vi "Get Physical DMA Address.vi"(8 "error in (no error)":errorcluster, 10 "Address2":u32, 11 "Address1":u32) -> (0 "error out":errorcluster, 1 "function return":u32, 2 "Address2 out":u32, 3 "Address1 out":u32)   [LabVIEW 2014, in "atmcd32d.lvlib"]
doc: "unsigned int WINAPI GetPhysicalDMAAddress(unsigned long * Address1, unsigned long * Address2);"
uses:
  atmcd32d.lvlib
  atmcd32d.dll
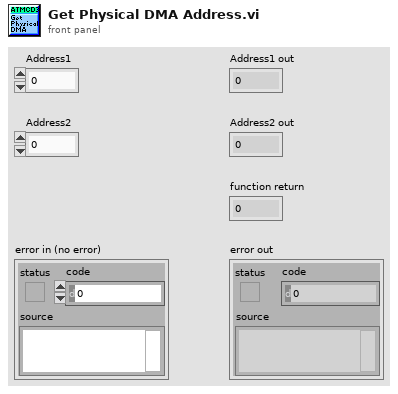
[diagram p1: front panel]
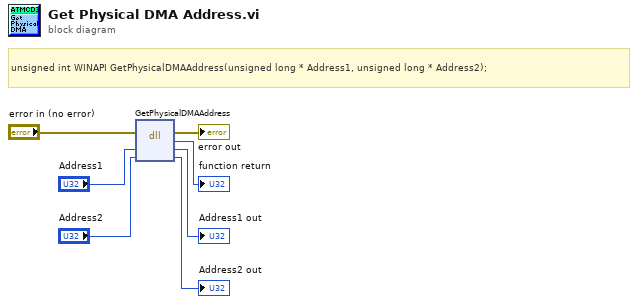
[diagram p0: block diagram]
diagram:
  # "unsigned int WINAPI GetPhysicalDMAAddress(unsigned long * Address1, unsigned long * Address2);"
  n1 = dll-call lib="C:/Users/Bakir/Documents/Lambda2-Testing/lib/Andorlib/atmcd32d.*" fn="GetPhysicalDMAAddress"(error in="error in (no error)", "Address1"="Address1", "Address2"="Address2") -> (error out=→"error out":errorcluster, →"function return":u32, "Address1"=→"Address1 out":u32, "Address2"=→"Address2 out":u32)  [unwired: 2 in, 1 out]
